vi "Execute.vi"(8 "error in (no error)":errorcluster, 9 "Workspace":T1, 10 "Cluster":T2={"I-O.lvclass"=refnum, "Motion.lvclass"=refnum, "Dispenser.lvclass"=refnum}, 11 "Pick and Place in":refnum<class "Pick and Place.lvclass">) -> (0 "error out":errorcluster, 2 "Control Out":T2, 3 "Pick and Place out":refnum<class "Pick and Place.lvclass">)   [LabVIEW 2016, in "Pick and Place.lvclass"]
uses:
  Pick and Place.lvclass
  Controller/Controllers.ctl
  Controller/I-O/I-O.lvclass
  Controller/Motion/A3200/A3200.lvclass
  Controller/Dispenser/Dispenser.lvclass
  Controller/Motion/Motion.lvclass
  Workspace/Workspace.ctl
  Pick and Place.lvclass/Pick and Place.ctl
  Controller/Controller.lvclass
  Workspace/Fixture.lvclass
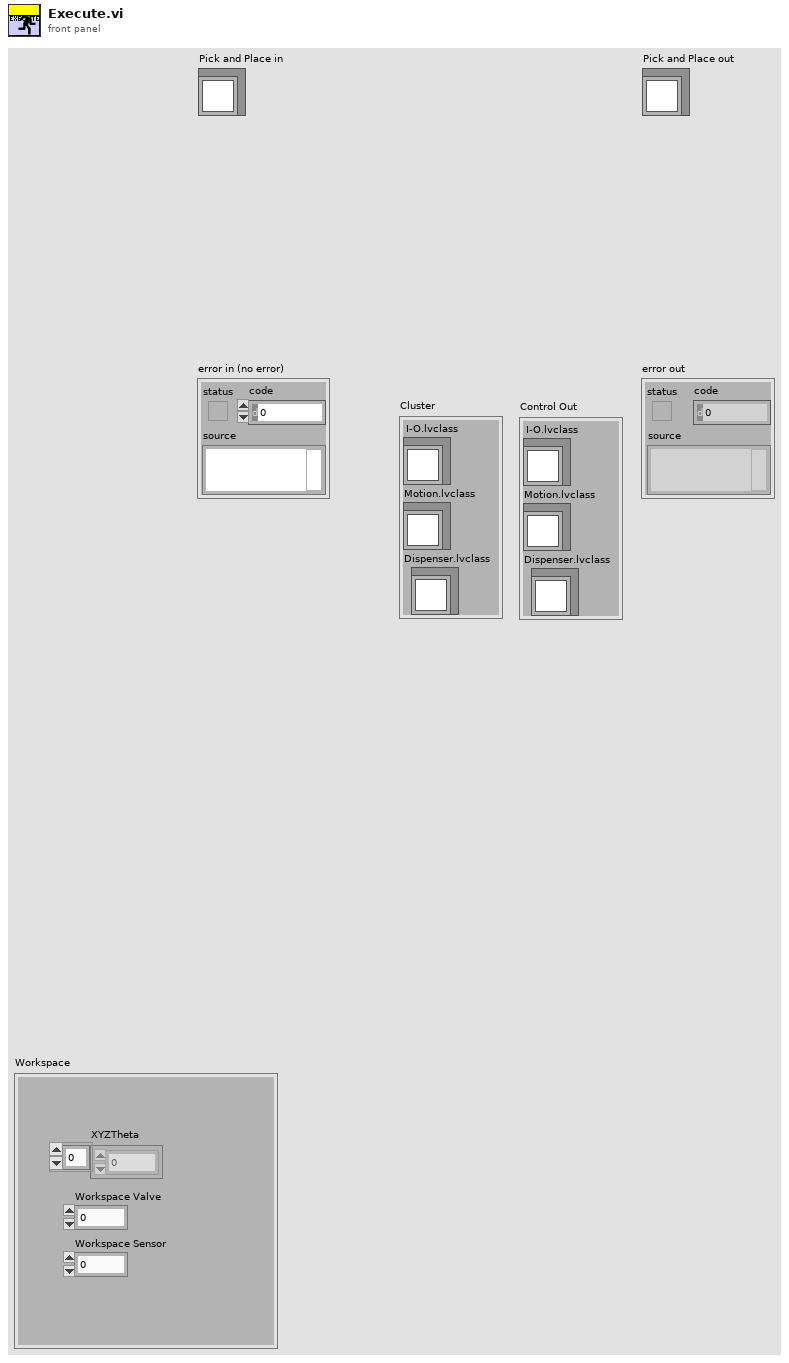
[diagram p1: front panel]
types:
  T1 = typedef "Fixture.lvclass/Workspace.ctl" = cluster{"XYZTheta":dbl[], "Workspace Valve":i32, "Workspace Sensor":i32}
  T2 = typedef "Controller.lvclass/Controllers.ctl" = cluster{"I-O.lvclass":refnum<class "I-O.lvclass">, "Motion.lvclass":refnum<class "Motion.lvclass">, "Dispenser.lvclass":refnum<class "Dispenser.lvclass">}
  T3 = typedef "Pick and Place.lvclass/Pick and Place Type.ctl" = enum16{"Primary Pick Up", "Secondary Pick Up", "Put Down All", "Pick Up All", "Put Down Secondary"}
  T4 = typedef "I-O.lvclass/Pin Map.ctl" = cluster{"Region Valves":i32[], "Extra Valves":dbl[][][], "Tool Primary Valve":i32, "Tool Secondary Valve":i32, "Region Sensors":i32[], "Extra Sensors":dbl[][][], "Tool Primary Sensor":dbl, "Tool Secondary Sensor":dbl, "Compression Sensor":dbl, "5V":i32}
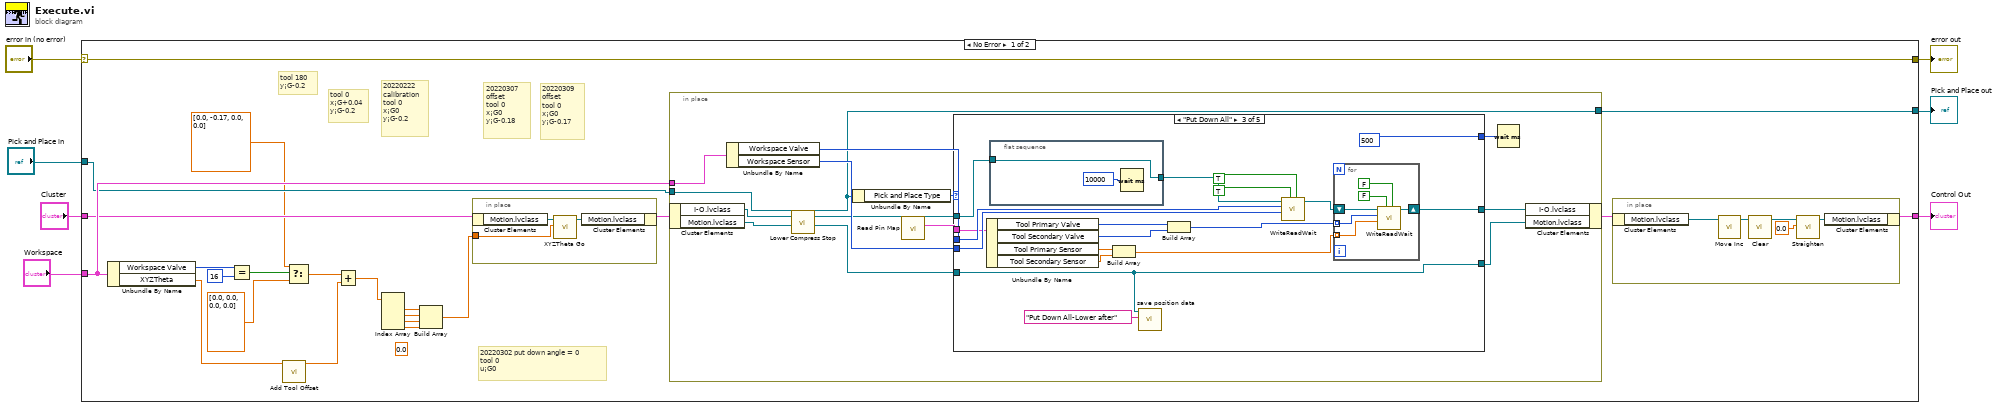
[diagram p0: block diagram]
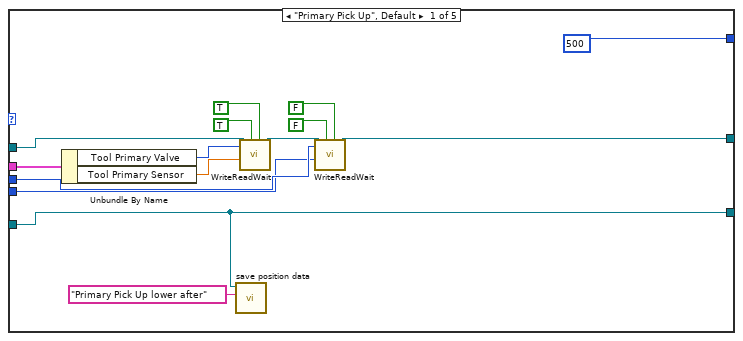
[diagram p2: hidden frame]
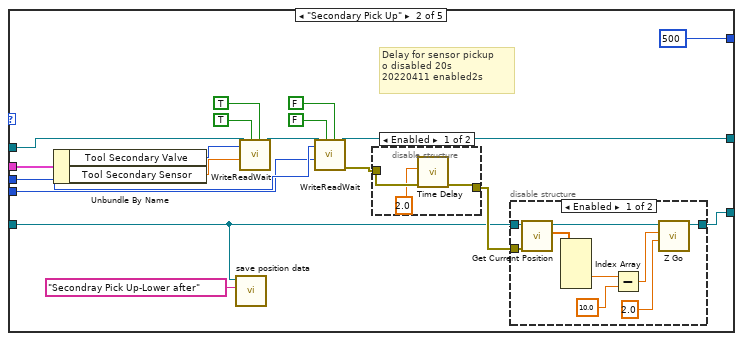
[diagram p3: hidden frame]
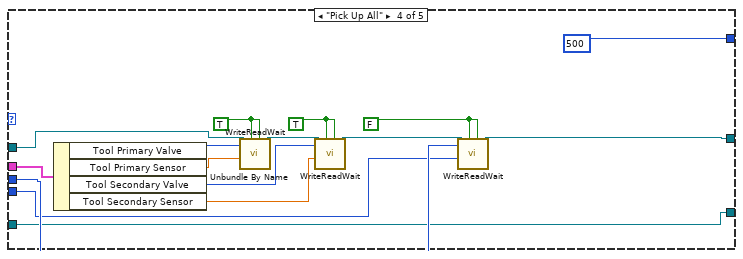
[diagram p6: hidden frame]
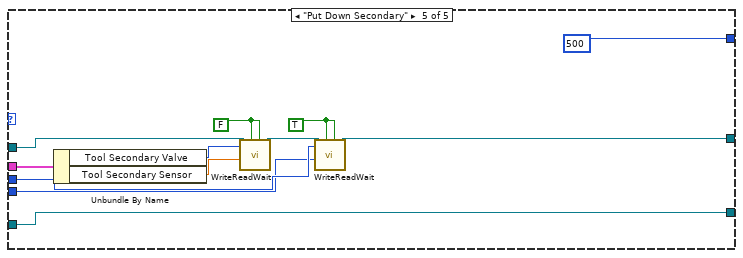
[diagram p7: hidden frame]
diagram:
  n1 = case shown="No Error" "error in (no error)" {
    selector: "error in (no error)" -> [w29 w155]
    tunnel: "Cluster" -> [w25 w156]
    tunnel: "Workspace" -> [w26 _]
    tunnel: [w29 w155] -> w1
    tunnel: [w24 w156] -> w2
    tunnel: "Pick and Place in" -> [w23 w154]
    tunnel: [w22 w154] -> w6
    frame No Error {
      (unwired) 0.0 ("element")
      # "20220309\noffset\ntool 0 \nx¡G0\ny¡G-0.17"
      # "20220307 \noffset\ntool 0 \nx¡G0\ny¡G-0.18"
      # "20220302 put down angle = 0\ntool 0\nu¡G0"
      # "20220222 \ncalibration\ntool 0 \nx¡G0\ny¡G-0.2"
      # "tool 180 \ny¡G-0.2"
      # "tool 0 \nx¡G+0.04\ny¡G-0.2"
      n2 = Unbundle By Name(w26) -> ("Workspace Valve"=w20:i32, "XYZTheta"=w21:dbl[])
      n3 = Equal?(x=w20, y=16) -> (x = y?=w18:bool)
      n4 = call "Add Tool Offset.vi"("XYZTheta"=w21) -> ("Array"=w16:dbl[])  [unwired: 10 in]
      n5 = Select(t=dbl[] [0.0, -0.17, 0.0, 0.0], s=w18, f=dbl[] [0.0, 0.0, 0.0, 0.0]) -> (s? t:f=w17:dbl[])
      n6 = Add(x=w17, y=w16) -> (x+y=w10:dbl[])
      n7 = Index Array(array=w10) -> (element #1=w11:dbl, element #2=w12:dbl, element #3=w13:dbl, element #4=w8:dbl)  [unwired: 4 in]
      n8 = Build Array(w11, w12, w13, w8) -> (w9:dbl[])
      n9 = in-place {
        in-place-border: w9 -> [w153]
        n10 = in-place-cluster #1(w25) -> ("Motion.lvclass"=w152:refnum<class "Motion.lvclass">)
        n11 = call "XYZTheta Go.vi"("XYZTheta In"=w153, "Motion in"=w152) -> ("Motion out"=w151:refnum<class "Motion.lvclass">)  [unwired: 7 in, 2 out]
        n12 = in-place-cluster #1("Motion.lvclass"=w151) -> (w28:T2)
      }
      n13 = in-place {
        in-place-border: w26 -> [w44]
        in-place-border: w23 -> [w33]
        in-place-border: [w32] -> w22
        n14 = in-place-cluster #2(w28) -> ("I-O.lvclass"=w37:refnum<class "I-O.lvclass">, "Motion.lvclass"=w36:refnum<class "Motion.lvclass">)
        n15 = Unbundle By Name(w44) -> ("Workspace Valve"=w42:i32, "Workspace Sensor"=w41:i32)
        n16 = call "Lower Compress Stop.vi"("Motion.lvclass"=w36, "I-O.lvclass"=w37, "Pick and Place in"=w33) -> ("Motion.lvclass"=w31:refnum<class "Motion.lvclass">, "I-O out"=w34:refnum<class "I-O.lvclass">, "Pick and Place Out"=w32:refnum<class "Pick and Place.lvclass">)  [unwired: 5 in, 1 out]
        n17 = Unbundle By Name(w32) -> ("Pick and Place Type"=w43:T3)
        n18 = call-dynamic "Read Pin Map.vi"("I-O in"=w34) -> ("Pin Map 2"=w39:T4, "I-O out"=w38:refnum<class "I-O.lvclass">)  [unwired: 8 in, 1 out]
        n19 = case shown="\"Put Down All\"" w43 {
          tunnel: w42 -> [w56 w69 w99 w123 w139]
          tunnel: w41 -> [w55 w68 w98 w122 w138]
          tunnel: [w50 w67 w103 w120 w136] -> w35
          tunnel: [u32 500 ("milliseconds to wait") 500 500 u32 500 ("milliseconds to wait") u32 500 ("milliseconds to wait")] -> w40
          tunnel: w38 -> [w49 w66 w94 w132 w144]
          tunnel: w39 -> [w48 w65 w97 w133 w145]
          tunnel: w31 -> [w45 w61 w92 w118 w134]
          tunnel: [w45 w63 w92 w118 w134] -> w30
          frame "Primary Pick Up", Default {
            n20 = Unbundle By Name(w48) -> ("Tool Primary Valve"=w47:i32, "Tool Primary Sensor"=w58:dbl)
            n21 = call "save position data.vi"("step name"="Primary Pick Up lower after", "Motion.lvclass"=w45) -> ()  [unwired: 9 in, 1 out]
            n22 = call "WriteReadWait.vi"("Read Value"=TRUE, "Write Value"=TRUE, "Read"=w58, "Write"=w47, "I-O in"=w49) -> ("I-O out"=w57:refnum<class "I-O.lvclass">)  [unwired: 5 in, 1 out]
            n23 = call "WriteReadWait.vi"("Read Value"=FALSE ("Write Value"), "Write Value"=FALSE ("Read Value"), "Read"=w55, "Write"=w56, "I-O in"=w57) -> ("I-O out"=w50:refnum<class "I-O.lvclass">)  [unwired: 5 in, 1 out]
          }
          frame "Secondary Pick Up" {
            # "Delay for sensor pickup\no disabled 20s\n20220411 enabled2s"
            n24 = Unbundle By Name(w65) -> ("Tool Secondary Valve"=w71:i32, "Tool Secondary Sensor"=w70:dbl)
            n25 = call "save position data.vi"("step name"="Secondray Pick Up-Lower after", "Motion.lvclass"=w61) -> ()  [unwired: 9 in, 1 out]
            n26 = call "WriteReadWait.vi"("Read Value"=TRUE, "Write Value"=TRUE, "Read"=w70, "Write"=w71, "I-O in"=w66) -> ("I-O out"=w76:refnum<class "I-O.lvclass">)  [unwired: 5 in, 1 out]
            n27 = call "WriteReadWait.vi"("Read Value"=FALSE ("Write Value"), "Write Value"=FALSE ("Read Value"), "Read"=w68, "Write"=w69, "I-O in"=w76) -> ("error out"=w64:errorcluster, "I-O out"=w67:refnum<class "I-O.lvclass">)  [unwired: 5 in]
            n28 = disable-structure shown="Enabled" {
              disable-tunnel: w64 -> [w80 w81]
              disable-tunnel: [w78 w81] -> w62
              frame Enabled {
                n29 = call "Time Delay"("error in (no error)"=w80, "Delay Time (s)"=2.0) -> ("error out"=w78:errorcluster)  [unwired: 9 in]
              }
              frame Disabled {
              }
            }
            n30 = disable-structure shown="Enabled" {
              disable-tunnel: [w89 w91] -> w63
              disable-tunnel: w61 -> [w88 w91]
              disable-tunnel: w62 -> [w87 _]
              frame Enabled {
                n31 = call-dynamic "Get Current Position.vi"("error in (no error)"=w87, "Motion in"=w88) -> ("XYZTheta Out"=w86:dbl[], "Motion out"=w90:refnum<class "Motion.lvclass">)  [unwired: 7 in, 1 out]
                n32 = Index Array(array=w86) -> (element #3=w85:dbl)  [unwired: 4 in, 3 out]
                n33 = Subtract(x=w85, y=10.0) -> (x-y=w84:dbl)
                n34 = call-dynamic "Z Go.vi"("Speed"=2.0, "Position"=w84, "Motion in"=w90) -> ("Motion out"=w89:refnum<class "Motion.lvclass">)  [unwired: 7 in, 1 out]
              }
              frame Disabled {
              }
            }
          }
          frame "Put Down All" {
            n35 = Unbundle By Name(w97) -> ("Tool Primary Valve"=w104:i32, "Tool Secondary Valve"=w105:i32, "Tool Primary Sensor"=w106:dbl, "Tool Secondary Sensor"=w107:dbl)
            n36 = flat-sequence {
              tunnel: [w110] -> w95
              tunnel: w94 -> [w110]
              frame #0 {
                # "Delay After Placing"
                n37 = Wait (ms)(milliseconds to wait=u32 10000) -> ()  [unwired: 1 out]
              }
            }
            n38 = Build Array(w106, w107) -> (w109:dbl[])
            n39 = call "save position data.vi"("step name"="Put Down All-Lower after", "Motion.lvclass"=w92) -> ()  [unwired: 9 in, 1 out]
            n40 = Build Array(w104, w105) -> (w108:i32[])
            n41 = call "WriteReadWait.vi"("Read Value"=TRUE, "Write Value"=TRUE, "Read"=w98, "Write"=w99, "I-O in"=w95) -> ("I-O out"=w96:refnum<class "I-O.lvclass">)  [unwired: 5 in, 1 out]
            n42 = for {
              shift-right: [w112] -> w103
              shift-left: w96 -> [w113]
              tunnel: w108 -> [w115] mode=indexing
              tunnel: w109 -> [w114] mode=indexing
              n43 = call "WriteReadWait.vi"("Read Value"=FALSE ("Write Value"), "Write Value"=FALSE ("Read Value"), "Read"=w114, "Write"=w115, "I-O in"=w113) -> ("I-O out"=w112:refnum<class "I-O.lvclass">)  [unwired: 5 in, 1 out]
            }
          }
          frame "Pick Up All" {
            w121 = FALSE ("Read Value")
            w125 = TRUE ("Write Value")
            w131 = TRUE ("Write Value")
            n44 = Unbundle By Name(w133) -> ("Tool Primary Valve"=w130:i32, "Tool Primary Sensor"=w129:dbl, "Tool Secondary Valve"=w127:i32, "Tool Secondary Sensor"=w126:dbl)
            n45 = call "WriteReadWait.vi"("Read Value"=w131, "Write Value"=w131, "Read"=w129, "Write"=w130, "I-O in"=w132) -> ("I-O out"=w128:refnum<class "I-O.lvclass">)  [unwired: 5 in, 1 out]
            n46 = call "WriteReadWait.vi"("Read Value"=w125, "Write Value"=w125, "Read"=w126, "Write"=w127, "I-O in"=w128) -> ("I-O out"=w124:refnum<class "I-O.lvclass">)  [unwired: 5 in, 1 out]
            n47 = call "WriteReadWait.vi"("Read Value"=w121, "Write Value"=w121, "Read"=w122, "Write"=w123, "I-O in"=w124) -> ("I-O out"=w120:refnum<class "I-O.lvclass">)  [unwired: 5 in, 1 out]
          }
          frame "Put Down Secondary" {
            w137 = TRUE ("Read Value")
            w141 = FALSE ("Write Value")
            n48 = Unbundle By Name(w145) -> ("Tool Secondary Valve"=w143:i32, "Tool Secondary Sensor"=w142:dbl)
            n49 = call "WriteReadWait.vi"("Read Value"=w141, "Write Value"=w141, "Read"=w142, "Write"=w143, "I-O in"=w144) -> ("I-O out"=w140:refnum<class "I-O.lvclass">)  [unwired: 5 in, 1 out]
            n50 = call "WriteReadWait.vi"("Read Value"=w137, "Write Value"=w137, "Read"=w138, "Write"=w139, "I-O in"=w140) -> ("I-O out"=w136:refnum<class "I-O.lvclass">)  [unwired: 5 in, 1 out]
          }
        }
        n51 = Wait (ms)(milliseconds to wait=w40) -> ()  [unwired: 1 out]
        n52 = in-place-cluster #2("I-O.lvclass"=w35, "Motion.lvclass"=w30) -> (w27:T2)
      }
      n53 = in-place {
        n54 = in-place-cluster #3(w27) -> ("Motion.lvclass"=w146:refnum<class "Motion.lvclass">)
        n55 = call-dynamic "Move Inc.vi"("Motion in"=w146) -> ("Motion out"=w147:refnum<class "Motion.lvclass">)  [unwired: 9 in, 1 out]
        n56 = call "Clear.vi"("Motion in"=w147) -> ("Motion out"=w150:refnum<class "Motion.lvclass">)  [unwired: 9 in, 1 out]
        n57 = call-dynamic "Straighten.vi"("Theta"=0.0 ("Angle (rad)"), "Motion in"=w150) -> ("Motion out"=w149:refnum<class "Motion.lvclass">)  [unwired: 8 in, 1 out]
        n58 = in-place-cluster #3("Motion.lvclass"=w149) -> (w24:T2)
      }
    }
    frame Error {
    }
  }
  "error out" <- w1
  "Pick and Place out" <- w6
  "Control Out" <- w2
